vi "List Databases.vi"(8 "error in (no error)":errorcluster, 10 "Context":string, 11 "mysql in":refnum<class "mysql.lvclass">) -> (0 "error out":errorcluster, 2 "databases":string[](array[string]), 3 "mysql out":refnum<class "mysql.lvclass">)   [LabVIEW 2020, in "mysql.lvlib" / "mysql.lvclass"]
uses:
  mysql.lvclass
  07ea7771-2020-4302-b487-6d62cae708c7.vi
  <vilib>/Utility/error.llb/Error Cluster From Error Code.vi
panel:
  out "database info":string[][](array[string])
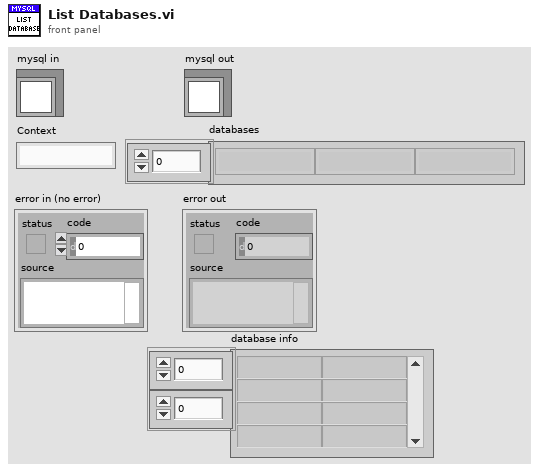
[diagram p1: front panel]
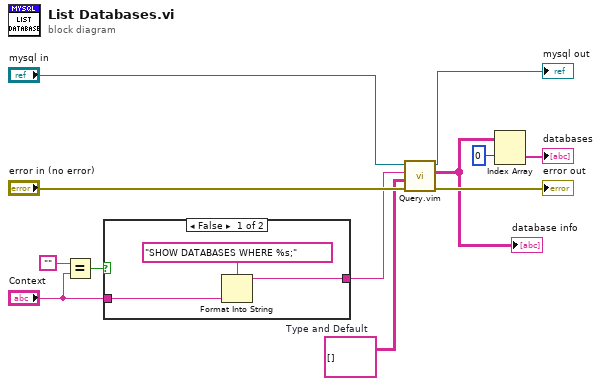
[diagram p0: block diagram]
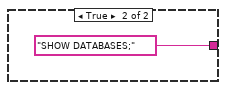
[diagram p2: hidden frame]
diagram:
  w1 = string[][] []  # Type and Default
  n1 = Equal?(x="", y="Context") -> (x = y?=w2:bool)
  n2 = case shown="False" w2 {
    tunnel: [w14 "SHOW DATABASES;" ("format string")] -> w5
    tunnel: "Context" -> [w13 _]
    frame False {
      n3 = Format Into String(format string="SHOW DATABASES WHERE %s;", w13) -> (resulting string=w14:string)  [unwired: 2 in, 1 out]
    }
    frame True {
    }
  }
  n4 = call "Query.vim"("error in (no error)"="error in (no error)", "Type and Default"=w1, "Query string"=w5, "IDatabase in"="mysql in") -> ("error out"=→"error out":errorcluster, "Result"=w6:string[][], "IDatabase out"=→"mysql out":refnum<class "mysql.lvclass">)  [unwired: 5 in]
  "database info" <- w6
  n5 = Index Array(array=w6, index (col)=0 ("disabled index (col)")) -> (element=→"databases":string[])  [unwired: 1 in]
